vi "Calculate Reynolds Number.vi"(6 "Q (lpm)":dbl, 7 "u (m/s)":dbl, 8 "ThroughPipe":bool, 9 "D (m)":dbl, 11 "T (degC)":dbl) -> (2 "u_out (m/s)":dbl, 3 "Re":dbl)   [LabVIEW 2016, in "Atmospheric Library.lvlib"]
uses:
  Atmospheric Library.lvlib
  Atmospheric Constants.vi
panel:
  out "mu (Pa*s)":dbl=1.4685620043524856e-05
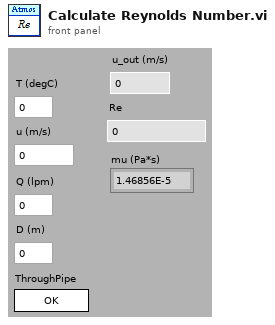
[diagram p1: front panel]
types:
  T1 = enum16{"Air", "N2", "O2", "CO2", "CO", "H2", "NH3", "SO2", "He"}
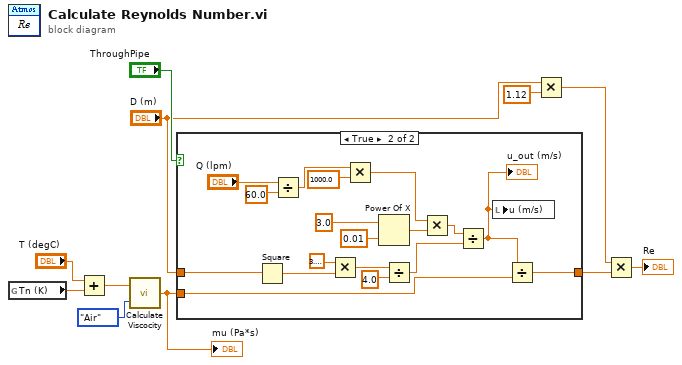
[diagram p0: block diagram]
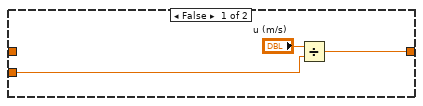
[diagram p2: hidden frame]
diagram:
  n1 = global read "Atmospheric Constants.vi" "Tn (K)"() -> (w10:dbl)
  n2 = Add(x="T (degC)", y=w10) -> (x+y=w9:dbl)
  n3 = call "Calculate Viscocity.vi"("Gas"=T1."Air", "T(K)"=w9) -> ("mu (Pa*s)"=w4:dbl)
  "mu (Pa*s)" <- w4
  n4 = case shown="True" "ThroughPipe" {
    tunnel: "D (m)" -> [_ w31]
    tunnel: w4 -> [w14 w16]
    tunnel: [w12 w21] -> w3
    frame False {
      n5 = Divide(x="u (m/s)", y=w14) -> (x/y=w12:dbl)
    }
    frame True {
      n6 = Square(x=w31) -> (x^2=w30:dbl)
      n7 = Divide(x="Q (lpm)", y=60.0) -> (x/y=w25:dbl)
      n8 = Multiply(x=3.141592653589793, y=w30) -> (x*y=w29:dbl)
      n9 = Multiply(x=w25, y=1000.0) -> (x*y=w23:dbl)
      n10 = Power Of X(1:0.01 ("y"), 2:3.0 ("x")) -> (0:w22:dbl)
      n11 = Divide(x=w29, y=4.0) -> (x/y=w17:dbl)
      n12 = Multiply(x=w23, y=w22) -> (x*y=w18:dbl)
      n13 = Divide(x=w18, y=w17) -> (x/y=w15:dbl)
      "u_out (m/s)" <- w15
      n14 = local write "u (m/s)"(w15) -> ()
      n15 = Divide(x=w15, y=w16) -> (x/y=w21:dbl)
    }
  }
  n16 = Multiply(x="D (m)", y=1.12) -> (x*y=w2:dbl)
  n17 = Multiply(x=w2, y=w3) -> (x*y=→"Re":dbl)
